vi "Send PUBREL.vi"(8 "error in (no error)":errorcluster, 10 "Message ID":u16=10 format="%x", 11 "connection ID":refnum<k5>) -> (0 "error out":errorcluster, 3 "connection ID out":refnum<k5>)   [LabVIEW 2020, in "DAQIO MQTT.lvlib"]
uses:
  DAQIO MQTT.lvlib
  Controls/MessageType.ctl
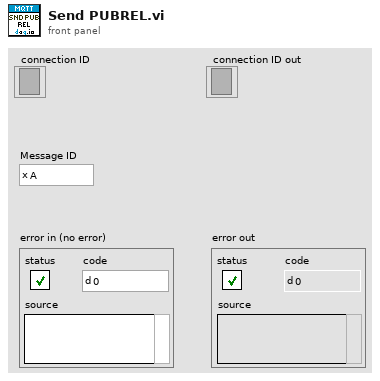
[diagram p1: front panel]
types:
  T1 = enum8{"At most once", "At least once", "Exactly once", "Reserved"}
  T2 = typedef "DAQIO MQTT.lvlib/MessageType.ctl" = enum32{"Reserved", "CONNECT", "CONNACK", "PUBLISH", "PUBACK", "PUBREC", "PUBREL", "PUBCOMP", "SUBSCRIBE", "SUBACK", "UNSUBSCRIBE", "UNSUBACK", "PINGREQ", "PINGRESP", "DISCONNECT", "Reserved2"}
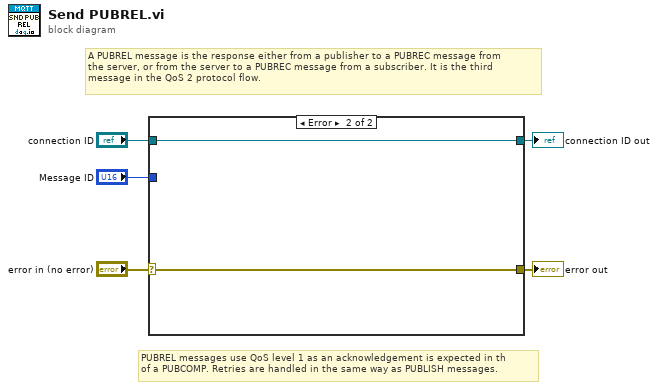
[diagram p0: block diagram]
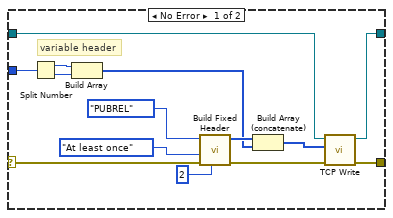
[diagram p2: hidden frame]
diagram:
  # "PUBREL messages use QoS level 1 as an acknowledgement is expected in th\nof a PUBCOMP. Retries are handled in the same way as PUBLISH messages."
  # "A PUBREL message is the response either from a publisher to a PUBREC message from\nthe server, or from the server to a PUBREC message from a subscriber. It is the third\nmessage in the QoS 2 protocol flow."
  n1 = case shown="Error" "error in (no error)" {
    selector: "error in (no error)" -> [w13 w21]
    tunnel: [w9 w21] -> w4
    tunnel: "connection ID" -> [w8 w20]
    tunnel: "Message ID" -> [w7 _]
    tunnel: [w6 w20] -> w1
    frame No Error {
      # "variable header"
      n2 = Split Number(x=w7) -> (hi(x)=w17:u8, lo(x)=w16:u8)
      n3 = Build Array(w17, w16) -> (w12:u8[])
      n4 = call "Build Fixed Header.vi"("Remaining Length"=u32 2, "error in (no error)"=w13, "QoS"=T1."At least once", "MessageType"=MessageType."PUBREL") -> ("error out"=w10:errorcluster, "Fixed Header"=w18:u8[])  [unwired: 6 in]
      n5 = Build Array (concatenate)(w18, w12) -> (w11:u8[])
      n6 = call "TCP Write.vi"("error in (no error)"=w10, "data in"=w11, "connection ID"=w8) -> ("error out"=w9:errorcluster, "connection ID out"=w6:refnum<k5>)  [unwired: 6 in, 1 out]
    }
    frame Error {
    }
  }
  "error out" <- w4
  "connection ID out" <- w1
